vi "DataToImage.vi"(6 "String":string, 7 "userID":string, 9 "Data in":string[][](array[string]), 10 "Boolean":bool, 11 "Refnum in":T1) -> (3 "Refnum out":T1)   [LabVIEW 2020]
uses:
  <vilib>/vision/Image Controls.llb/IMAQ Image.ctl
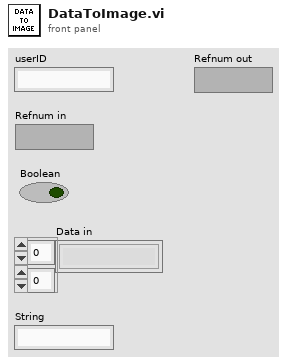
[diagram p1: front panel]
types:
  T1 = typedef "IMAQ Image.ctl" = refnum<image>
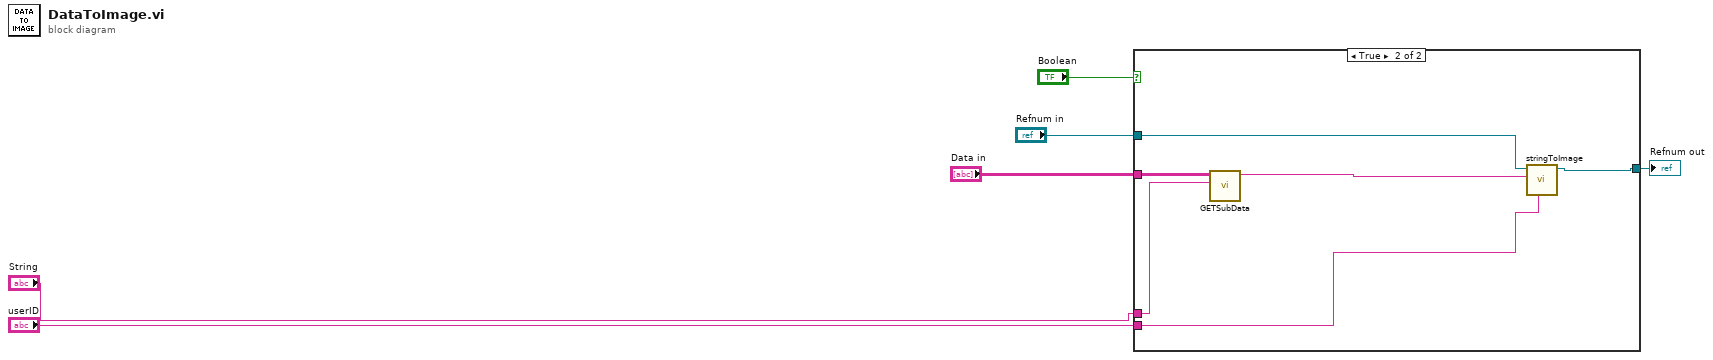
[diagram p0: block diagram]
diagram:
  n1 = case shown="True" "Boolean" {
    tunnel: "Data in" -> [_ w13]
    tunnel: "String" -> [_ w10]
    tunnel: "userID" -> [_ w11]
    tunnel: "Refnum in" -> [w7 w9]
    tunnel: [w7 w8] -> w6
    frame False {
    }
    frame True {
      n2 = call "GETSubData.vi"("Variable Header"=w10, "Data out"=w13) -> ("delimiter (Tab)"=w12:string)  [unwired: 9 in]
      n3 = call "stringToImage.vi"("label text (image name)"=w11, "data in"=w12, "Refnum in"=w9) -> ("Refnum out"=w8:T1)  [unwired: 5 in, 3 out]
    }
  }
  "Refnum out" <- w6
